vi "Programm 1.vi"() -> ()   [LabVIEW 2020]
panel:
  in  "Format-String":string
  in  "Dateipfad (Dialog verwenden)":path=path "C:/Users/Messlabor_Kustos/Desktop/test.xls"
  in  "Numerisches Element":dbl
  out "Numerisches Anzeigeelement":dbl
  out "Signalverlaufsdiagramm":dynamicdata(graph)
  in  "Stopp":bool
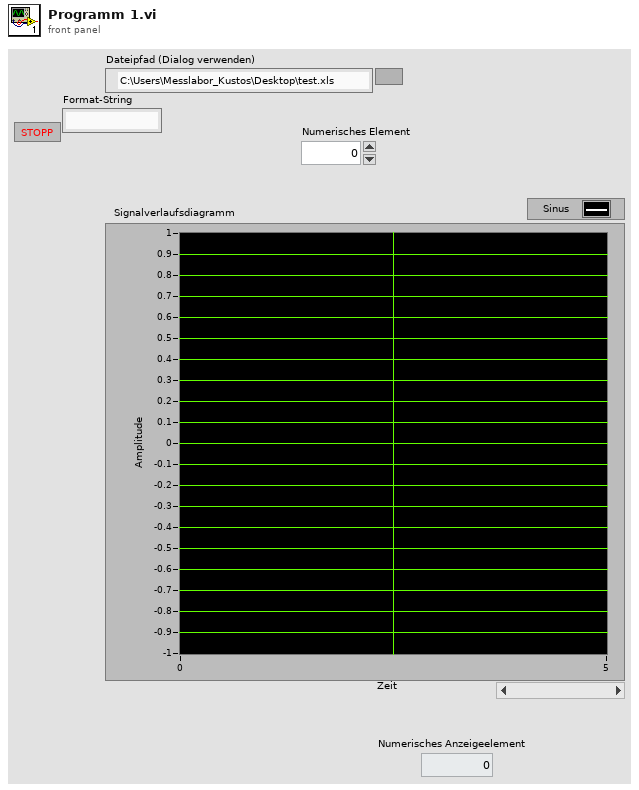
[diagram p1: front panel]
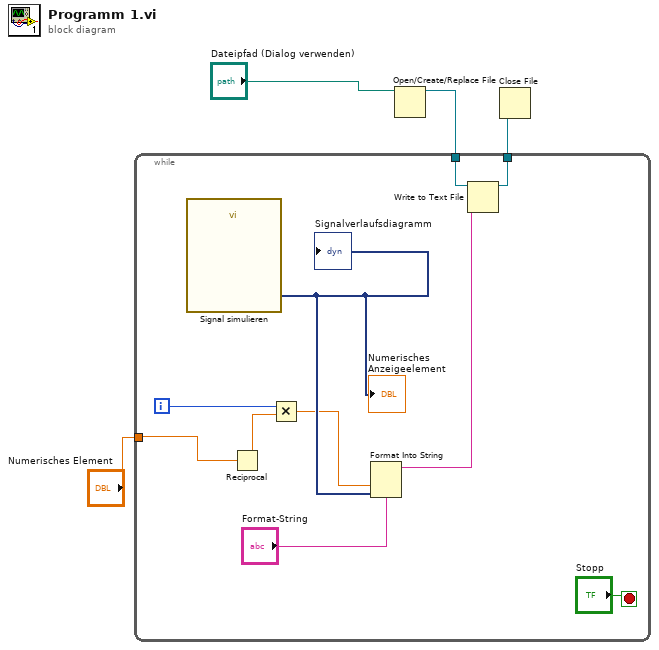
[diagram p0: block diagram]
diagram:
  n1 = Open/Create/Replace File(file path (use dialog)="Dateipfad (Dialog verwenden)") -> (refnum out=w1:refnum<file>)  [unwired: 5 in, 2 out]
  n2 = while {
    tunnel: "Numerisches Element" -> [w13]
    tunnel: [w8] -> w3
    tunnel: w1 -> [w7]
    i -> [w6]
    stop <- "Stopp" stop-if-true
    n3 = call "Signal simulieren"() -> ("Sinus"=w11:dynamicdata)  [unwired: 14 in, 1 out]
    "Signalverlaufsdiagramm" <- w11
    "Numerisches Anzeigeelement" <- w11
    n4 = Reciprocal(x=w13) -> (1/x=w12:dbl)
    n5 = Multiply(x=w6, y=w12) -> (x*y=w10:dbl)
    n6 = Format Into String(format string="Format-String", w10, w11) -> (resulting string=w9:string)  [unwired: 2 in, 1 out]
    n7 = Write to Text File(file (use dialog)=w7, text=w9) -> (refnum out=w8:refnum<file>)  [unwired: 2 in, 2 out]
  }
  n8 = Close File(refnum=w3) -> ()  [unwired: 1 in, 2 out]
